vi "Append Hypertext Link Anchor to Report.vi"(0 "report in":refnum<class "NI_Standard Report.lvclass">, 1 "MS Office parameters":T1, 5 "URL of link - href":string, 9 "link text":string, 11 "error in (no error)":errorcluster) -> (4 "report out":refnum<class "NI_Standard Report.lvclass">, 8 "start out (Word)":i32, 10 "end out (Word)":i32, 15 "error out":errorcluster)   [LabVIEW 2020, in "NI_Standard Report.lvclass"]
doc: "Creates and adds a hypertext link anchor to a Word, Excel, or HTML report. You cannot use this VI with standard reports."
uses:
  <vilib>/Utility/NIReport.llb/Standard Report/NI_Standard Report.lvclass
  <vilib>/Utility/NIReport.llb/NI_ReportGenerationCore.lvlib
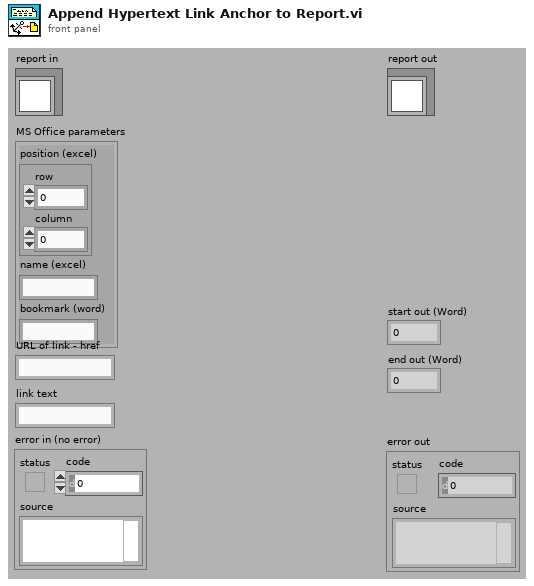
[diagram p1: front panel]
types:
  T1 = cluster{"position (excel)":cluster{"row":i32, "column":i32}, "name (excel)":string, "bookmark (word)":string}
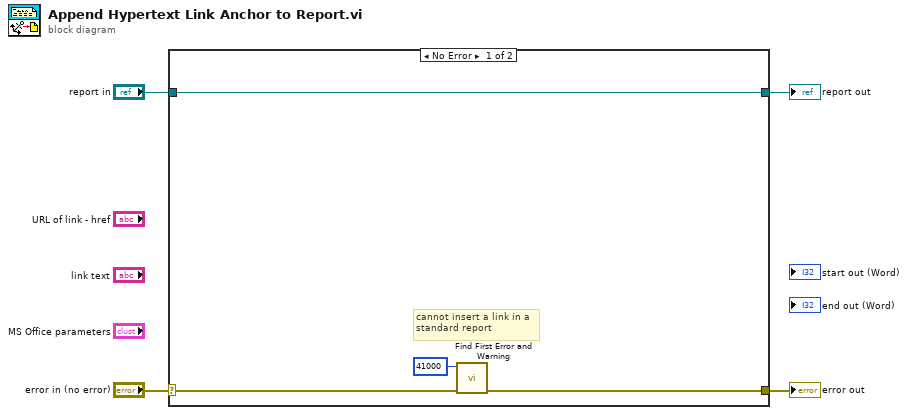
[diagram p0: block diagram]
diagram:
  n1 = case shown="No Error" "error in (no error)" {
    selector: "error in (no error)" -> [w6 w10]
    tunnel: [w5 w10] -> w3
    tunnel: [w8 w9] -> w1
    tunnel: "report in" -> [w8 w9]
    frame No Error {
      # "cannot insert a link in a\nstandard report"
      n2 = call <vilib>:"Find First Error and Warning.vi"("error in (no error)"=w6, "error code"=41000) -> ("error out"=w5:errorcluster)  [unwired: 1 in, 4 out]
    }
    frame Error {
    }
  }
  "error out" <- w3
  "report out" <- w1
